vi "WLM Control.vi"(8 "error in (no error)":errorcluster, 10 "command":enum16{"show", "hide", "exit"}(ring)) -> (0 "error out":errorcluster, 2 "return value":u32)   [LabVIEW 2017]
doc: "Show, hides, or exits the wavelength meter (WLM) server. If the server is not running, and either show or hide are called, it will start."
uses:
  <vilib>/Utility/error.llb/DialogType.ctl
  HighFinesse WS5/wlmData.dll
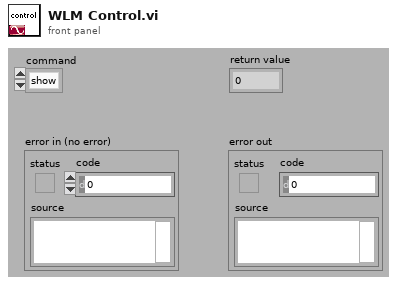
[diagram p1: front panel]
types:
  T1 = typedef "DialogType.ctl" = u16
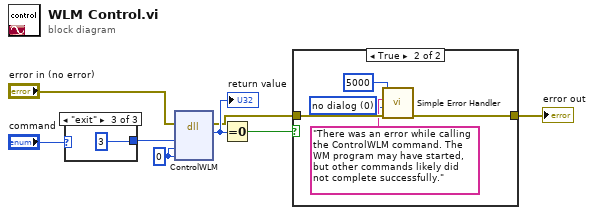
[diagram p0: block diagram]
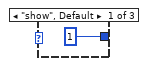
[diagram p3: hidden frame]
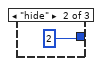
[diagram p4: hidden frame]
diagram:
  w8 = 0 ("Res1")
  n1 = case shown="\"exit\"" "command" {
    tunnel: [1 ("Res1") 2 ("Res1") 3 ("Res1")] -> w6
    frame "show", Default {
    }
    frame "hide" {
    }
    frame "exit" {
    }
  }
  n2 = dll-call lib="C:/LabVIEW-programs-dev/Instruments/Wavelength meter/HighFinesse WS5/wlmData.dll" fn="ControlWLM"(error in="error in (no error)", "Action"=w6, "App"=w8, "Res1"=w8) -> (error out=w3:errorcluster, "return type"=w5:u32)  [unwired: 5 in, 1 out]
  "return value" <- w5
  n3 = Equal To 0?(x=w5) -> (x = 0?=w4:bool)
  n4 = case shown="True" w4 {
    tunnel: w3 -> [w12 w17]
    tunnel: [w12 w14] -> w1
    frame False {
    }
    frame True {
      w15 = T1 0 items=["no dialog", "OK message", "continue or stop message", "OK message + warnings", "continue/stop + warnings"] ("type of dialog (OK msg:1)")
      n5 = call <vilib>:"Simple Error Handler.vi"("error code (no error:0)"=5000, "error source (\" \")"="There was an error while calling the ControlWLM command. The WM program may have started, but other commands likely did not complete successfully." ("error source (\" \")"), "type of dialog (OK msg:1)"=w15, "error in (no error)"=w17) -> ("error out"=w14:errorcluster)  [unwired: 5 out]
    }
  }
  "error out" <- w1
